vi "3D01_Basic_Plot_3D_Data.vi"() -> ()   [LabVIEW 2012]
uses:
  <vilib>/Utility/miscctls.llb/LVRangeTypeDef.ctl
  <userlib>/Photonfocus Toolkit/_Public/SubVIs/pf_Set_Camera_Property_Float.vi
  <userlib>/Photonfocus Toolkit/_Public/SubVIs/pf_Set_Camera_Property_Mode.vi
  <userlib>/Photonfocus Toolkit/Photonfocus_Toolkit.lvlib
panel:
  in  "stop":bool
  out "Slide":i32(slide) scale=0.0..500.0
  in  "Tab Control":T1(tab)
  in  "Interface Name":string="img0::0||port0"
  in  "Profiles No.":i32=500
  out "Peak":sgl[](graph)
  out "Image":T2(plugin-control)
  out "Width":sgl[](graph)
  out "Quality":u8[](graph)
  out "Quality":T2(plugin-control)
  out "Range":T2(plugin-control)
  out "Width":T2(plugin-control)
  in  "3D Surface":refnum<k7>(container)
  in  "Range Min":sgl=200.0
  # "1 - Open MAX and specify the correct .icd file."
  # "2 - Get the interface name from MAX (e.g: \"imag0\") and write it in the following text field. \n\n3 - Add \"::\" and the Port number showed in MAX.\n\n4 - Add \"||\" and the port name showed in PFRemote."
  # "::"
  # "||port0"
  # "Example:   img0::0||port0"
  # "5 - Close MAX before start grabbing"
  # "Points corresponding to Range values below \"Range Min\" will be not plotted."
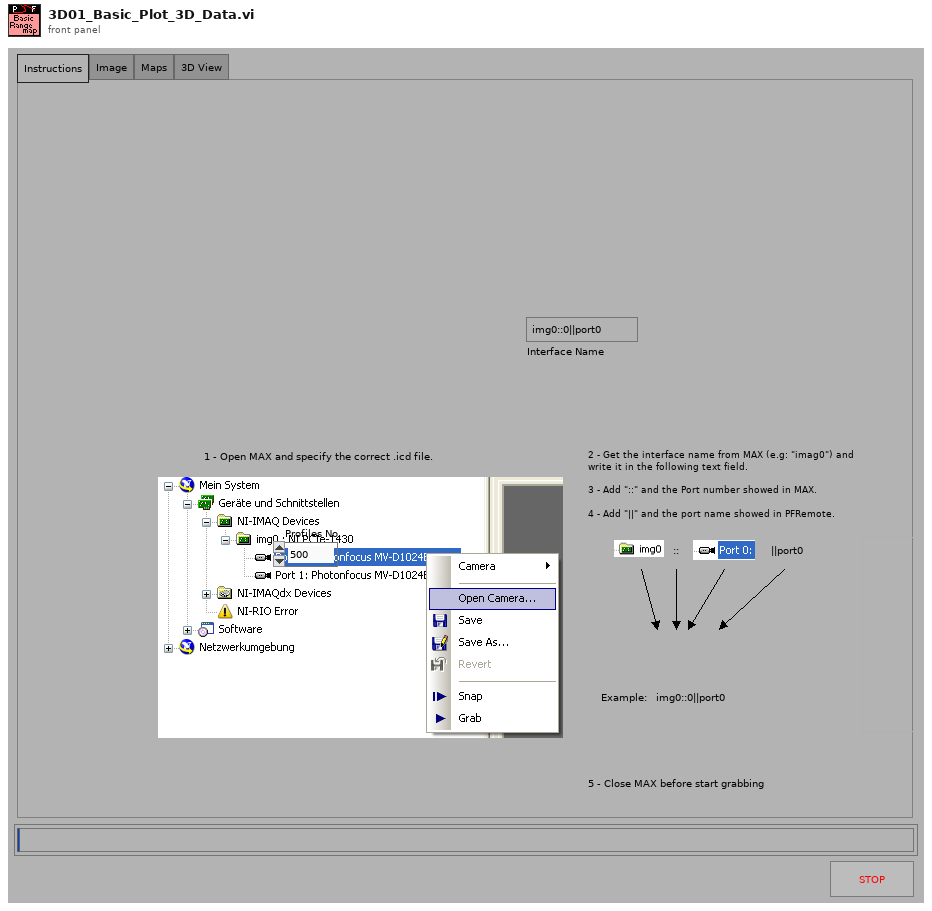
[diagram p1: front panel]
types:
  T1 = enum32{"Instructions", "Image", "Maps", "3D View"}
  T2 = typedef "IMAQ Image.ctl" = refnum<image>
  T3 = typedef "Image Type" = u32
  T4 = typedef "LVRangeTypeDef.ctl" = cluster{"Minimum":dbl, "Maximum":dbl, "Increment":dbl, "Minor Increment":dbl, "Start":dbl}
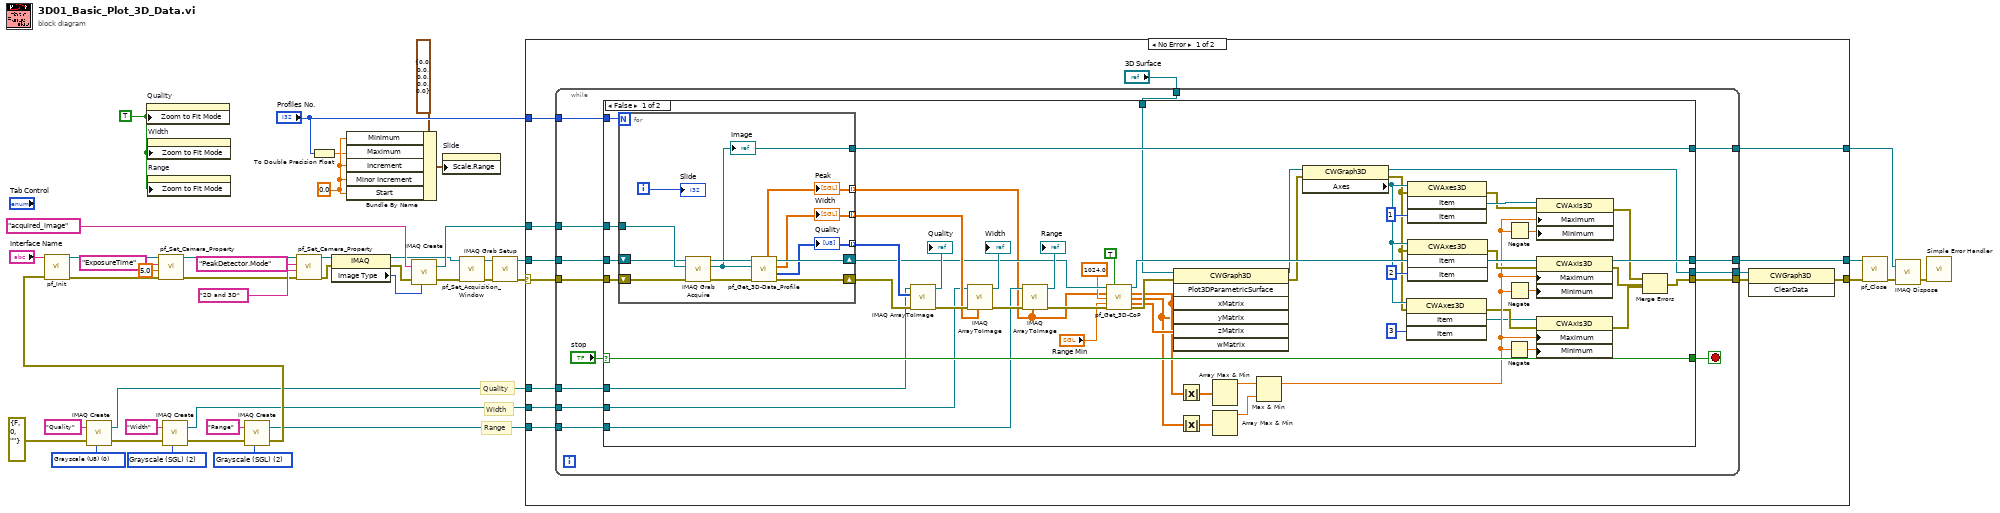
[diagram p0: block diagram]
diagram:
  w1 = TRUE ("Zoom to Fit Mode")
  w2 = T3 2 items=["Grayscale (U8)", "Grayscale (I16)", "Grayscale (SGL)", "Complex (CSG)", "RGB (U32)", "HSL (U32)", "RGB (U64)", "Grayscale (U16)"] ("Image Type")
  w6 = T3 2 items=["Grayscale (U8)", "Grayscale (I16)", "Grayscale (SGL)", "Complex (CSG)", "RGB (U32)", "HSL (U32)", "RGB (U64)", "Grayscale (U16)"] ("Image Type")
  w7 = T3 0 items=["Grayscale (U8)", "Grayscale (I16)", "Grayscale (SGL)", "Complex (CSG)", "RGB (U32)", "HSL (U32)", "RGB (U64)", "Grayscale (U16)"] ("Image Type")
  w16 = 0.0 ("Start")
  # "Quality"
  # "Width"
  # "Range"
  n1 = call "IMAQ Create"("Image Name"="Quality", "Image Type"=w7, "error in (no error)"=errorcluster {"status"=FALSE, "code"=0, "source"=""}) -> ("New Image"=w5:T2, "error out"=w14:errorcluster)  [unwired: 1 in, 1 out]
  n2 = property on="Quality" class="ImageControl"("Zoom to Fit Mode"=w1) -> ()  [unwired: 2 in, 2 out]
  n3 = property on="Width" class="ImageControl"("Zoom to Fit Mode"=w1) -> ()  [unwired: 2 in, 2 out]
  n4 = property on="Range" class="ImageControl"("Zoom to Fit Mode"=w1) -> ()  [unwired: 2 in, 2 out]
  n5 = call "IMAQ Create"("Image Name"="Width", "Image Type"=w2, "error in (no error)"=w14) -> ("New Image"=w4:T2, "error out"=w13:errorcluster)  [unwired: 1 in, 1 out]
  n6 = call "IMAQ Create"("Image Name"="Range", "Image Type"=w6, "error in (no error)"=w13) -> ("New Image"=w3:T2, "error out"=w8:errorcluster)  [unwired: 1 in, 1 out]
  n7 = call <userlib>:"pf_Init.vi"("error in (no error)"=w8, "Interface Name"="Interface Name") -> ("error out"=w22:errorcluster, "IMAQ Session out"=w20:refnum<k11>)  [unwired: 1 in, 7 out]
  n8 = call-poly <userlib>:"pf_Set_Camera_Property.vi"("error in (no error)"=w22, "Property Value"=sgl 5.0, "Property Name"="ExposureTime", "IMAQ Session in"=w20) -> ("error out"=w21:errorcluster, "IMAQ Session out"=w19:refnum<k11>)  [unwired: 6 out]
  n9 = call-poly <userlib>:"pf_Set_Camera_Property.vi"("error in (no error)"=w21, "Property Value"="2D and 3D", "Property Name"="PeakDetector.Mode", "IMAQ Session in"=w19) -> ("error out"=w27:errorcluster, "IMAQ Session out"=w28:refnum<k11>)  [unwired: 6 out]
  n10 = To Double Precision Float(number="Profiles No.") -> (double precision float=w15:dbl)
  n11 = property class="IMAQ"(reference=w28, error in=w27) -> (reference out=w26:refnum<k11>, error out=w44:errorcluster, "Image Type"=w45:u32)
  n12 = Bundle By Name(cluster=T4 {"Minimum"=0.0, "Maximum"=0.0, "Increment"=0.0, "Minor Increment"=0.0, "Start"=0.0} ("Scale.Range"), "Minimum"=w16, "Maximum"=w15, "Increment"=w16, "Minor Increment"=w16, "Start"=w16) -> (w23:T4)
  n13 = call "IMAQ Create"("Image Name"="acquired_image", "Image Type"=w45, "error in (no error)"=w44) -> ("New Image"=w31:T2, "error out"=w43:errorcluster)  [unwired: 1 in, 1 out]
  n14 = property on="Slide" class="Slide (strict)"("Scale.Range"=w23) -> ()  [unwired: 2 in, 2 out]
  n15 = call <userlib>:"pf_Set_Acquisition_Window.vi"("error in (no error)"=w43, "IMAQ Session in"=w26) -> ("error out"=w42:errorcluster, "IMAQ Session out"=w37:refnum<k11>)  [unwired: 8 out]
  n16 = call <vilib>:"IMAQ Grab Setup.vi"("error in (no error)"=w42, "IMAQ Session In"=w37) -> ("error out"=w32:errorcluster, "IMAQ Session Out"=w34:refnum<k11>)  [unwired: 8 out]
  n17 = case shown="No Error" w32 {
    selector: w32 -> [w55 w147]
    tunnel: [w46 w147] -> w36
    tunnel: w31 -> [w58 w146]
    tunnel: [w57 w146] -> w39
    tunnel: w34 -> [w56 w145]
    tunnel: [w54 w145] -> w33
    tunnel: "Profiles No." -> [w53 _]
    tunnel: w5 -> [w52 _]
    tunnel: w4 -> [w51 _]
    tunnel: w3 -> [w50 _]
    frame No Error {
      n18 = while {
        tunnel: w58 -> [w72]
        tunnel: [w71] -> w57
        tunnel: w56 -> [w70]
        tunnel: w55 -> [w69]
        tunnel: [w68] -> w54
        tunnel: [w67] -> w48
        tunnel: w53 -> [w66]
        tunnel: w52 -> [w63]
        tunnel: w51 -> [w62]
        tunnel: w50 -> [w61]
        tunnel: "3D Surface" -> [w60]
        tunnel: [w59] -> w47
        stop <- w64 stop-if-true
        n19 = case shown="False" "stop" {
          selector: "stop" -> [w122 w144]
          tunnel: w72 -> [w127 w141]
          tunnel: [w126 w141] -> w71
          tunnel: w70 -> [w125 w143]
          tunnel: w69 -> [w124 w142]
          tunnel: [w108 w143] -> w68
          tunnel: [w81 w142] -> w67
          tunnel: w66 -> [w123 _]
          tunnel: [w122 w144] -> w64
          tunnel: w63 -> [w113 _]
          tunnel: w62 -> [w112 _]
          tunnel: w61 -> [w111 _]
          tunnel: w60 -> [w102 w140]
          tunnel: [w98 w140] -> w59
          frame False {
            n20 = for {
              N: w123 -> [_]
              tunnel: w127 -> [w139]
              tunnel: [w137] -> w126
              shift-right: [w135] -> w121
              shift-left: w124 -> [w129]
              shift-right: [w134] -> w109
              shift-left: w125 -> [w128]
              tunnel: [w133] -> w101 mode=indexing
              tunnel: [w132] -> w118 mode=indexing
              tunnel: [w131] -> w117 mode=indexing
              i -> [w130]
              n21 = call <vilib>:"IMAQ Grab Acquire.vi"("error in (no error)"=w129, "Image In"=w139, "IMAQ Session In"=w128) -> ("error out"=w136:errorcluster, "Image Out"=w137:T2, "IMAQ Session Out"=w138:refnum<k11>)  [unwired: 1 in, 5 out]
              "Image" <- w137
              n22 = call <userlib>:"pf_Get_3D-Data_Profile.vi"("error in (no error)"=w136, "Aquired Image"=w137, "IMAQ Session in"=w138) -> ("error out"=w135:errorcluster, "Quality Profile"=w132:u8[], "Width Profile"=w131:sgl[], "IMAQ Session out"=w134:refnum<k11>, "Peak Profile"=w133:sgl[])  [unwired: 2 in, 2 out]
              "Peak" <- w133
              "Width" <- w131
              "Quality" <- w132
              "Slide" <- w130
            }
            n23 = call "IMAQ ArrayToImage"("error in (no error)"=w121, "Image Pixels (U8)"=w118, "Image"=w113) -> ("error out"=w120:errorcluster, "Image Out"=→"Quality":T2)  [unwired: 3 in, 4 out]
            n24 = call "IMAQ ArrayToImage"("Image Pixels (Float)"=w117, "error in (no error)"=w120, "Image"=w112) -> ("error out"=w119:errorcluster, "Image Out"=→"Width":T2)  [unwired: 3 in, 4 out]
            n25 = call "IMAQ ArrayToImage"("Image Pixels (Float)"=w101, "error in (no error)"=w119, "Image"=w111) -> ("error out"=w110:errorcluster, "Image Out"=→"Range":T2)  [unwired: 3 in, 4 out]
            n26 = call <userlib>:"pf_Get_3D-CoP.vi"("IMAQ Session in"=w109, "Truncate Range"=TRUE, "Range Map in"=w101, "Range Max"=sgl 1024.0, "Range Min"="Range Min", "error in (no error)"=w110) -> ("IMAQ Session out"=w108:refnum<k11>, "X Matrix"=w91:sgl[][], "Y Matrix"=w90:sgl[][], "Z Matrix"=w106:sgl[][], "error out"=w107:errorcluster)  [unwired: 2 in, 3 out]
            n27 = invoke class="CWGraph3D" method="Plot3DParametricSurface"(reference=w102, error in=w107, "xMatrix"=w91, "yMatrix"=w90, "zMatrix"=w106) -> (reference out=w100:refnum<k7>, error out=w99:errorcluster)  [unwired: 2 in, 5 out]
            n28 = Absolute Value(x=w91) -> (abs(x)=w89:sgl[][])
            n29 = Absolute Value(x=w90) -> (abs(x)=w88:sgl[][])
            n30 = Array Max & Min(array=w89) -> (max value=w87:sgl)  [unwired: 3 out]
            n31 = Array Max & Min(array=w88) -> (max value=w86:sgl)  [unwired: 3 out]
            n32 = Max & Min(x=w87, y=w86) -> (max(x,y)=w78:sgl)  [unwired: 1 out]
            n33 = property class="CWGraph3D"(reference=w100, error in=w99) -> (reference out=w98:refnum<k7>, error out=w75:errorcluster, "Axes"=w80:refnum<k7>)
            n34 = invoke class="CWAxes3D" method="Item"(reference=w80, error in=w75, "Item"=3) -> (error out=w74:errorcluster, "Item"=w73:refnum<k7>)  [unwired: 1 in, 2 out]
            n35 = invoke class="CWAxes3D" method="Item"(reference=w80, error in=w75, "Item"=1) -> (error out=w93:errorcluster, "Item"=w96:refnum<k7>)  [unwired: 1 in, 2 out]
            n36 = invoke class="CWAxes3D" method="Item"(reference=w80, error in=w75, "Item"=2) -> (error out=w92:errorcluster, "Item"=w95:refnum<k7>)  [unwired: 1 in, 2 out]
            n37 = Negate(x=w78) -> (-x=w77:sgl)
            n38 = Negate(x=w78) -> (-x=w84:sgl)
            n39 = Negate(x=w78) -> (-x=w85:sgl)
            n40 = property class="CWAxis3D"(reference=w95, error in=w92, "Maximum"=w78, "Minimum"=w85) -> (error out=w82:errorcluster)  [unwired: 1 out]
            n41 = property class="CWAxis3D"(reference=w73, error in=w74, "Maximum"=w78, "Minimum"=w77) -> (error out=w76:errorcluster)  [unwired: 1 out]
            n42 = property class="CWAxis3D"(reference=w96, error in=w93, "Maximum"=w78, "Minimum"=w84) -> (error out=w83:errorcluster)  [unwired: 1 out]
            n43 = Merge Errors(w83, w82, w76) -> (w81:errorcluster)
          }
          frame True {
          }
        }
      }
      n44 = invoke class="CWGraph3D" method="ClearData"(reference=w47, error in=w48) -> (error out=w46:errorcluster)  [unwired: 1 in, 2 out]
    }
    frame Error {
    }
  }
  n45 = call <userlib>:"pf_Close.vi"("error in (no error)"=w36, "IMAQ Session in"=w33) -> ("error out"=w35:errorcluster)  [unwired: 9 out]
  n46 = call "IMAQ Dispose"("Image"=w39, "error in (no error)"=w35) -> ("error out"=w41:errorcluster)  [unwired: 1 in, 3 out]
  n47 = call <vilib>:"Simple Error Handler.vi"("error in (no error)"=w41) -> ()  [unwired: 1 in, 8 out]
